vi "C867_Init.vi"(8 "error in":errorcluster caption="entrée d'erreur") -> (0 "error out":errorcluster caption="sortie d'erreur")   [LabVIEW 2026]
uses:
  Controls/TypeDef_FGV.ctl
  C867-VIs/Low Level/PI_GCS2_DLL_x64.dll
panel:
  in  "nBaudRate":i32=115200
  in  "nPortNr":i32=15
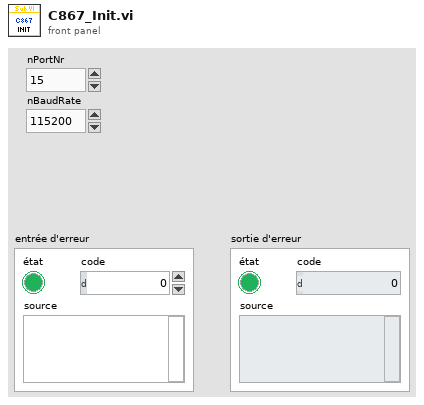
[diagram p1: front panel]
types:
  T1 = typedef "TypeDef_FGV.ctl" = enum16{"Initialize", "Write", "Read"}
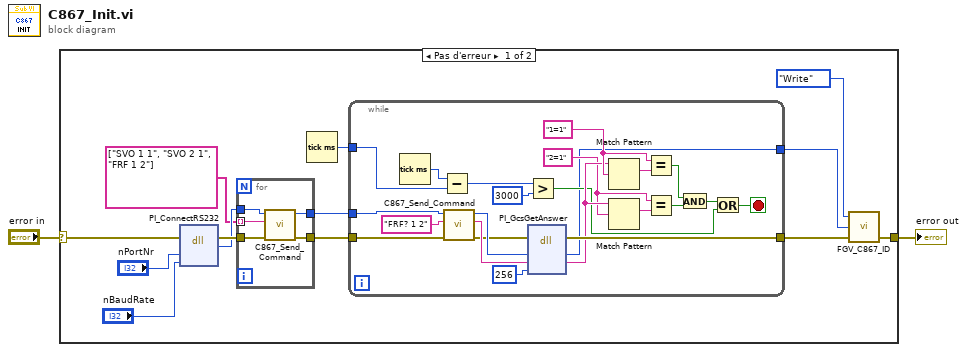
[diagram p0: block diagram]
diagram:
  n1 = case shown="Pas d'erreur" "error in" {
    selector: "error in" -> [w15 w44]
    tunnel: [w5 w44] -> w1
    frame No Error {
      n2 = dll-call lib="C:/Users/Sebastien/Documents/GitHub/LABVIEW-Useful-codes/Device_control/PC-C867-IO Control/v0.1/SubVI/PI-C867/C867-VIs/Low Level/PI_GCS2_DLL_x64.dll" fn="PI_ConnectRS232"(error in=w15, "nPortNr"="nPortNr", "nBaudRate"="nBaudRate") -> (error out=w14:errorcluster, "ID"=w9:i32)  [unwired: 4 in, 1 out]
      n3 = for {
        tunnel: string[] ["SVO 1 1", "SVO 2 1", "FRF 1 2"] -> [w16] mode=indexing
        tunnel: w14 -> [w20]
        tunnel: [w18] -> w8
        tunnel: w9 -> [w19]
        tunnel: [w17] -> w7
        n4 = call "C867_Send_Command.vi"("entrée d'erreur (pas d'erreur)"=w20, "szCommand"=w16, "ID en entrée"=w19) -> ("sortie d'erreur"=w18:errorcluster, "ID en sortie"=w17:i32)  [unwired: 6 in, 1 out]
      }
      n5 = Tick Count (ms)() -> (millisecond timer value=w11:u32)
      n6 = while {
        tunnel: w8 -> [w26]
        tunnel: w7 -> [w24]
        tunnel: [w43] -> w4
        tunnel: w11 -> [w40]
        tunnel: [w27] -> w3
        stop <- w30 stop-if-true
        w33 = "2=1" ("chaîne recherchée")
        w37 = "1=1" ("chaîne recherchée")
        n7 = Tick Count (ms)() -> (millisecond timer value=w41:u32)
        n8 = Subtract(x=w41, y=w40) -> (x-y=w39:u32)
        n9 = call "C867_Send_Command.vi"("entrée d'erreur (pas d'erreur)"=w26, "szCommand"="FRF? 1 2", "ID en entrée"=w24) -> ("sortie d'erreur"=w21:errorcluster, "szCommand out"=w23:string, "ID en sortie"=w22:i32)  [unwired: 6 in]
        n10 = Greater?(x=w39, y=u32 3000) -> (0:w31:bool)
        n11 = dll-call lib="C:/Users/Sebastien/Documents/GitHub/LABVIEW-Useful-codes/Device_control/PC-C867-IO Control/v0.1/SubVI/PI-C867/C867-VIs/Low Level/PI_GCS2_DLL_x64.dll" fn="PI_GcsGetAnswer"(error in=w21, "ID"=w22, "buffer"=w23, "buffersize"=256) -> (error out=w43:errorcluster, "ID"=w27:i32, "buffer"=w35:string)  [unwired: 4 in, 1 out]
        n12 = Match Pattern(string=w35, regular expression=w37) -> (match substring=w36:string)  [unwired: 1 in, 3 out]
        n13 = Match Pattern(string=w35, regular expression=w33) -> (match substring=w34:string)  [unwired: 1 in, 3 out]
        n14 = Equal?(x=w37, y=w36) -> (x = y?=w29:bool)
        n15 = Equal?(x=w33, y=w34) -> (x = y?=w28:bool)
        n16 = And(x=w29, y=w28) -> (x .and. y?=w32:bool)
        n17 = Or(x=w32, y=w31) -> (x .or. y?=w30:bool)
      }
      n18 = call "FGV_C867_ID.vi"("error in"=w4, "ID"=w3, "Action"=TypeDef_FGV."Write") -> ("error out"=w5:errorcluster)  [unwired: 1 in, 1 out]
    }
    frame Error {
    }
  }
  "error out" <- w1
